vi "09_dosing.vi"() -> ()   [LabVIEW 2024]
uses:
  <vilib>/Utility/error.llb/DialogType.ctl
  4067e6f5-c9bb-441e-8d38-abed3cce061a.vi
  <vilib>/Waveform/WDTOps.llb/WDT Get XY Value DBL.vi
  <vilib>/Utility/file.llb/Write Delimited Spreadsheet (DBL).vi
  <instrlib>/Tektronix DMM40x0 Series/Tektronix DMM40x0 Series.lvlib
panel:
  out "Current Time":timestamp
  out "Current Voltage":dbl format="%0.2f"
  in  "stop":bool
  out "STABLE":bool
  in  "Serial Communication":T1={"Baud Rate"=9600, "Parity"=0, "Data Bits"=8, "Stop Bits"=10, "Flow Control"=0} {"Flow Control" items=["None", "XON/XOFF", "RTS/CTS", "XON/XOFF & RTS/CTS", "DTR/DSR", "XON/XOFF & DTR/DSR"]; "Stop Bits" items=["1.0"=10, "1.5"=15, "2.0"=20]; "Data Bits" items=["7"=7, "8"=8]; "Parity" items=["None", "Odd", "Even", "Mark", "Space"]; "Baud Rate" items=["300"=300, "600"=600, "1200"=1200, "2400"=2400, "4800"=4800, "9600"=9600, "19200"=19200]}
  out "Stability threshold":dbl format="%#_13g"
  out "Waveform Graph":dbl[](graph)
  # "Voltmeter Serial Configuration"
  # "DEFAULT SETTINGS:\n\nTimeout (10000 ms)\nTrigger Count (5000)\nSample Count (1)\n\n****DC VOLTAGE***"
  # "Voltmeter Stability"
  # "0 - Stability threshold not met\n1 - Stability threshold met\n\n\n\n*stability (+/-0.05 mV) of last 15 pts"
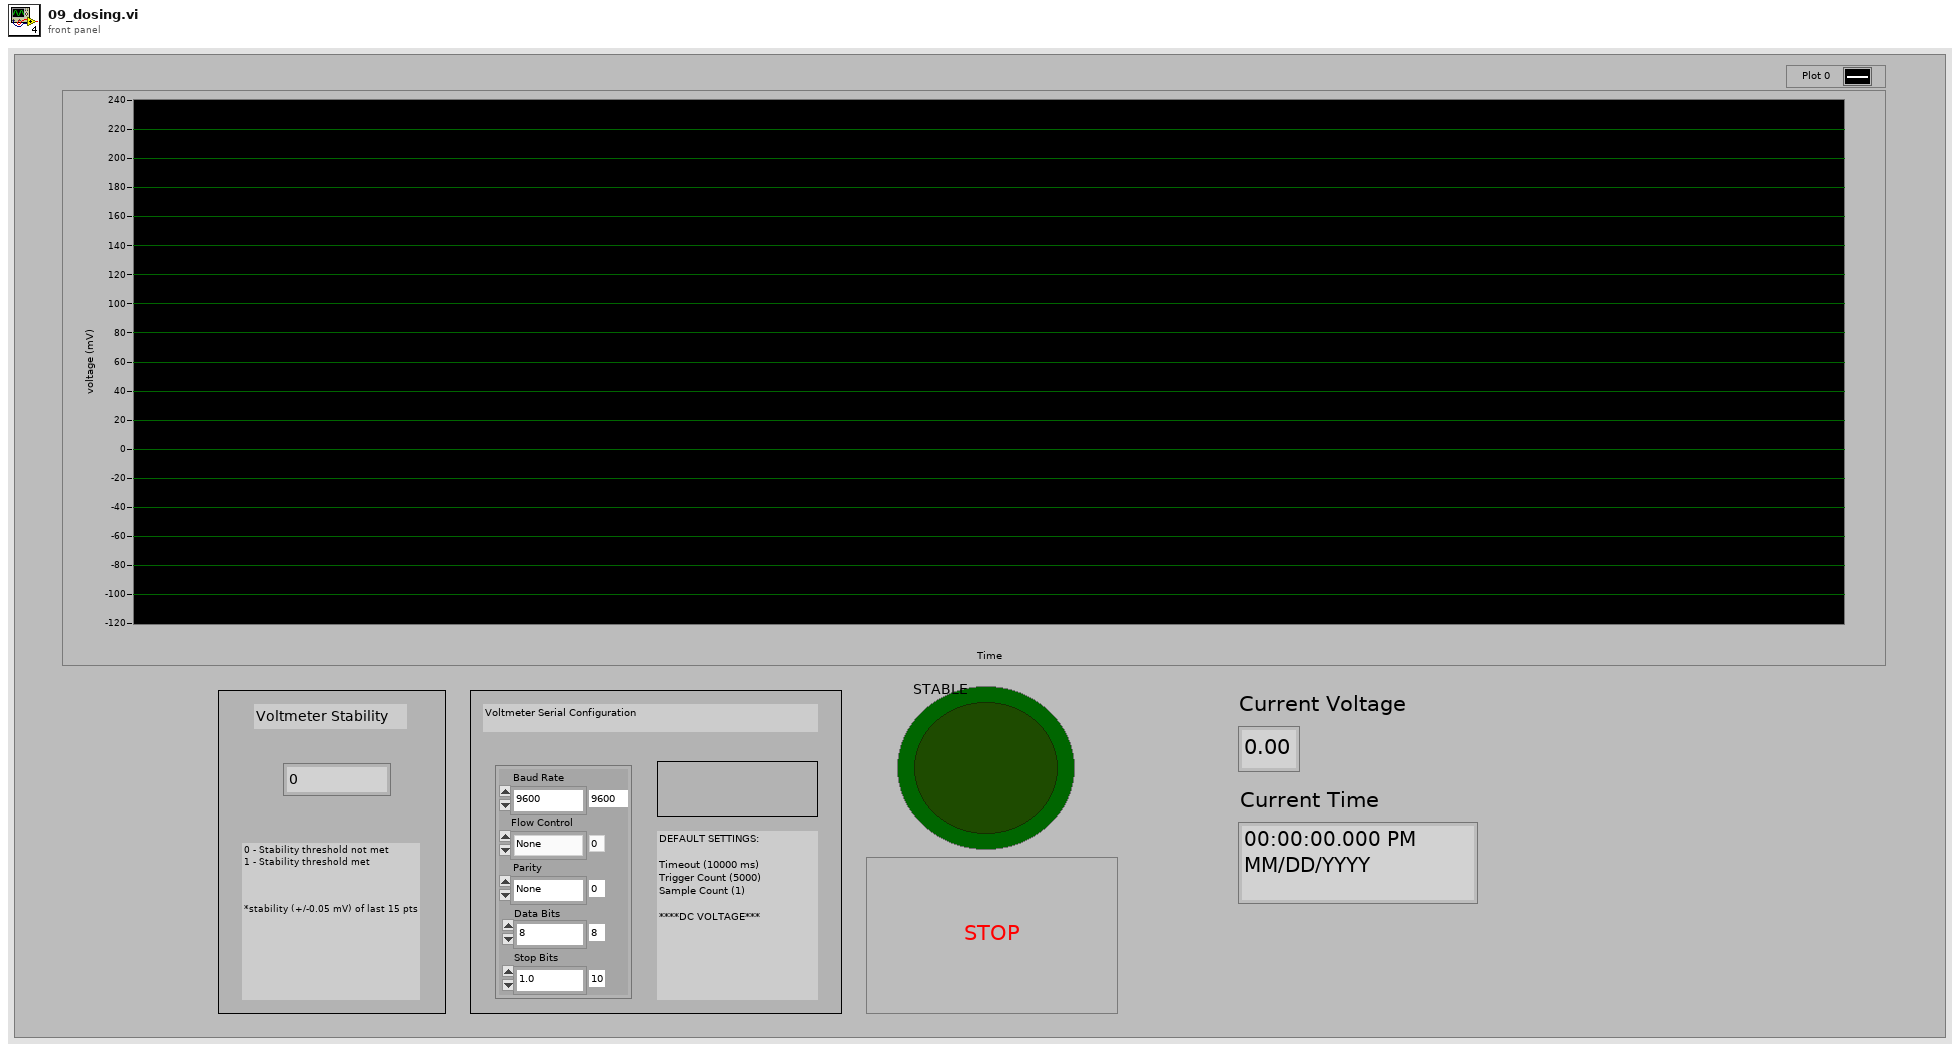
[diagram p1: front panel]
types:
  T1 = cluster{"Baud Rate":u32, "Parity":u16, "Data Bits":u16, "Stop Bits":u16, "Flow Control":u16}
  T2 = typedef "DialogType.ctl" = u16
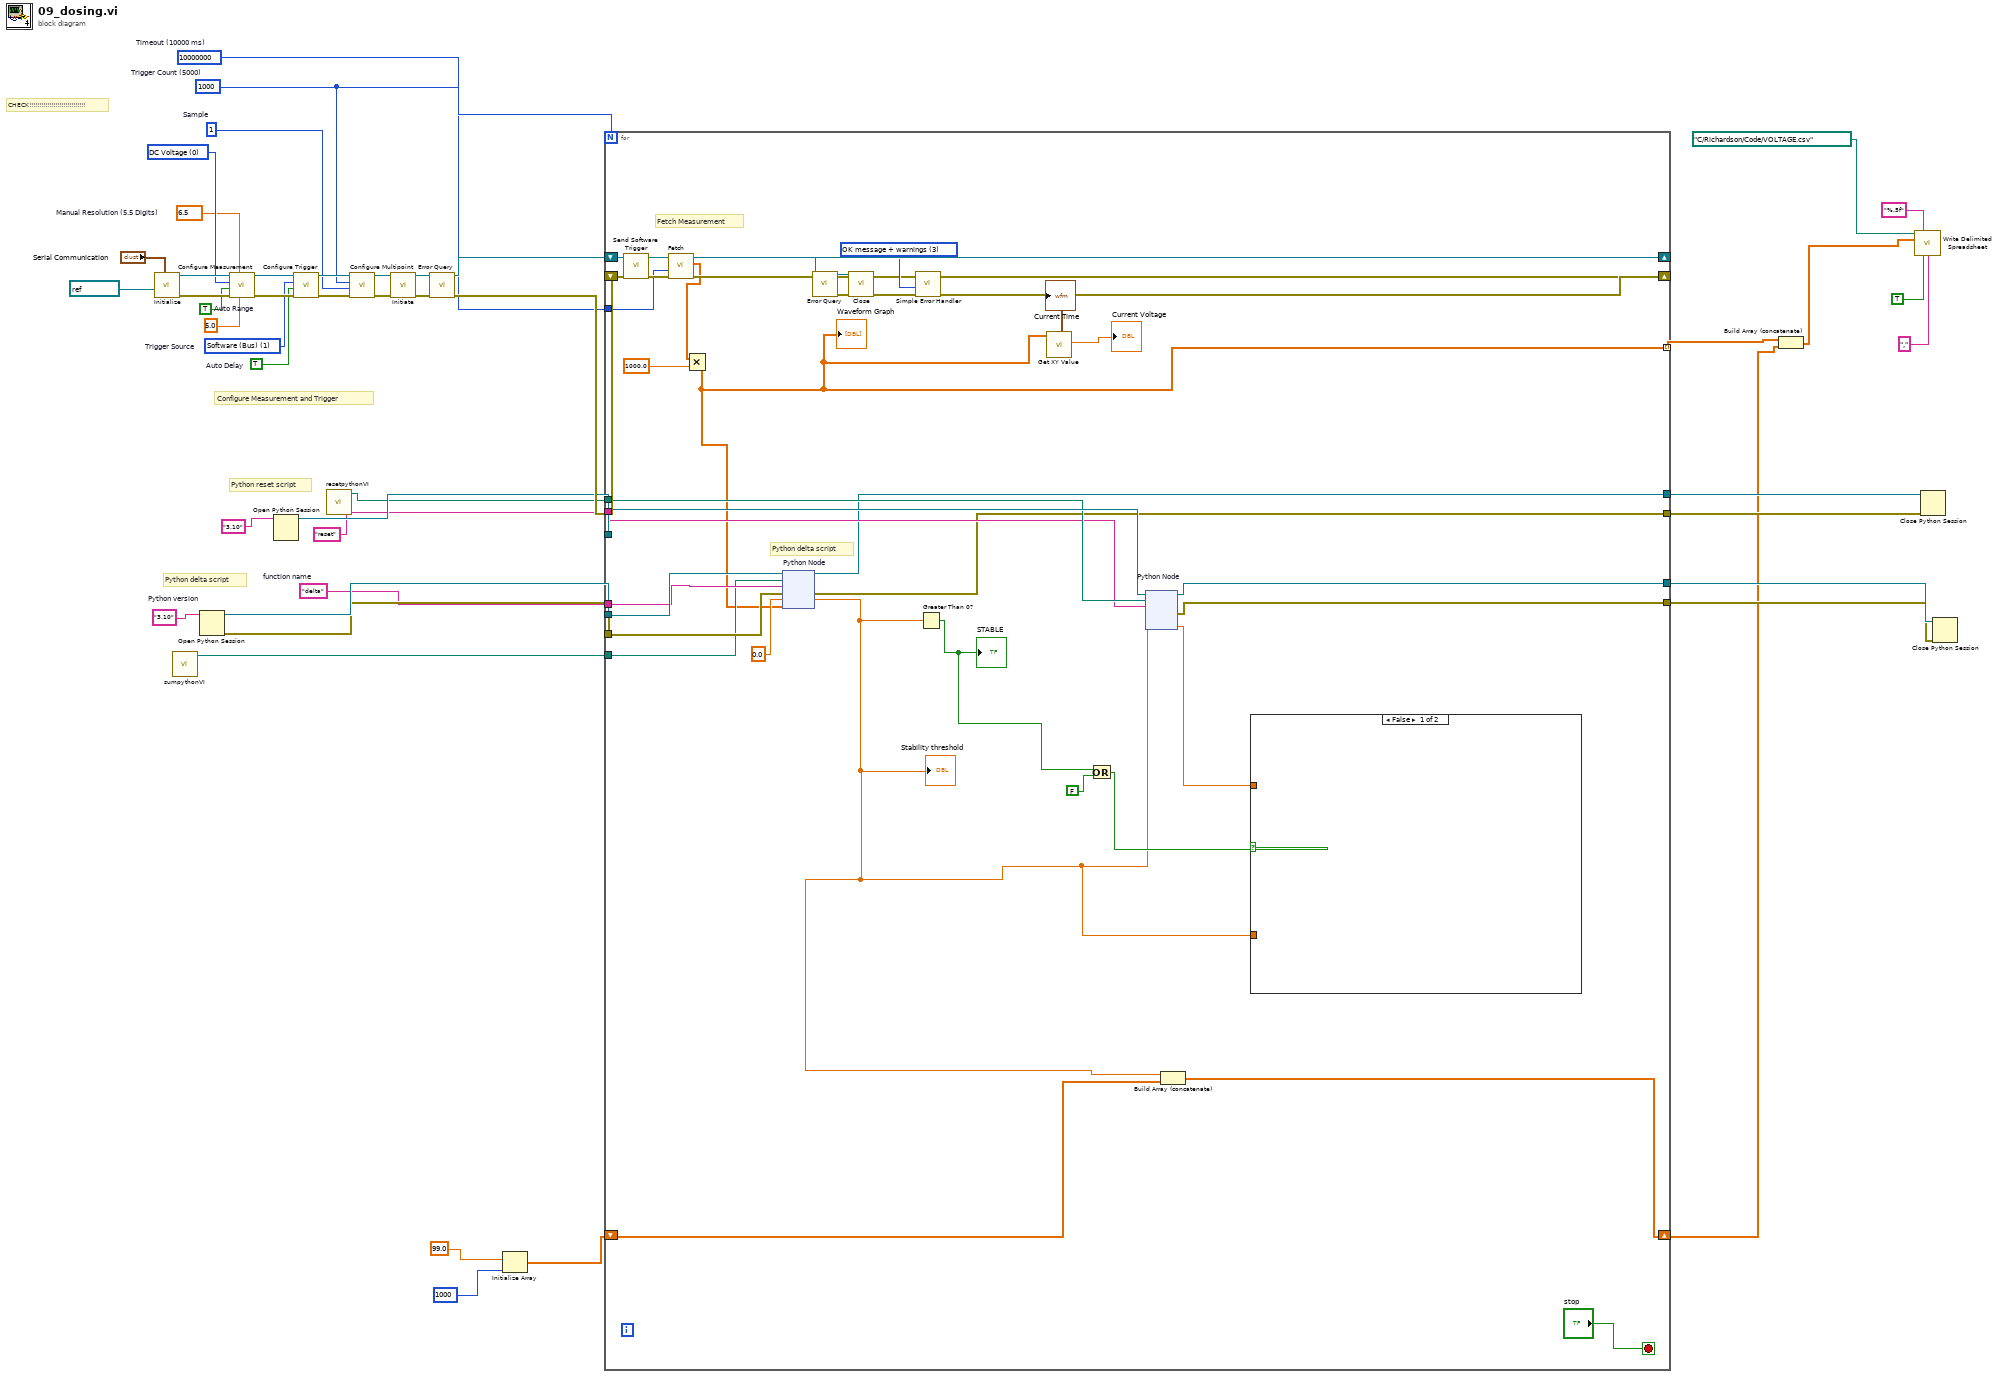
[diagram p0: block diagram]
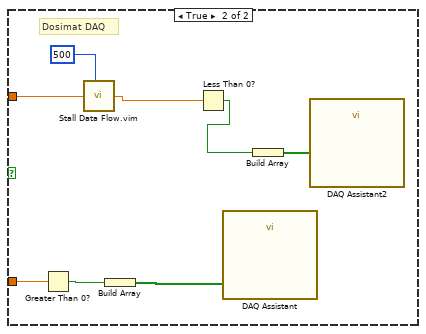
[diagram p2: hidden frame]
diagram:
  w11 = T2 3 items=["no dialog", "OK message", "continue or stop message", "OK message + warnings", "continue/stop + warnings"] ("type of dialog (OK msg:1)")
  w24 = "delta"  # function name
  w27 = "3.10"  # Python version
  w39 = u16 0 items=["DC Voltage", "AC Voltage", "2 - Wire Resistance", "4 - Wire Resistance", "DC Current", "AC Current", "Frequency", "Period", "Continuity", "Diode Checking", "Temperature", "Capacitance"] ("Function (0: DC Voltage)")
  w30 = u32 10000000  # Timeout (10000 ms)
  w31 = 1  # Sample
  w38 = 1000  # Trigger Count (5000)
  w32 = 6.5 items=["4.5"=4.5, "5.5"=5.5, "6.5"=6.5]  # Manual Resolution (5.5 Digits)
  w40 = TRUE  # Auto Delay
  w41 = u16 1 items=["Immediate", "Software (Bus)", "External"]  # Trigger Source
  w42 = TRUE  # Auto Range
  # "Python delta script"
  # "Python reset script"
  # "CHECK!!!!!!!!!!!!!!!!!!!!!!!!!!!!"
  # "Configure Measurement and Trigger"
  n1 = call <instrlib>:"Initialize.vi"("Serial Configuration"="Serial Communication", "VISA resource name"=refnum<visa-resource-name> "COM2" ("COM PORT (COM2)")) -> ("error out"=w51:errorcluster, "VISA resource name out"=w52:refnum<visa-resource-name>)  [unwired: 3 in, 5 out]
  n2 = call "sumpythonVI.vi"() -> ("appended path"=w23:path)  [unwired: 11 in]
  n3 = Open Python Session(python version=w27) -> (session out=w29:refnum<k35>, error out=w28:errorcluster)  [unwired: 2 in]
  n4 = call <instrlib>:"Configure Measurement.vi"("Manual Range (1.0)"=5.0, "Manual Resolution (5.5 Digits)"=w32, "error in (no error)"=w51, "Auto Range (T:Enable)"=w42, "Function (0: DC Voltage)"=w39, "VISA resource name"=w52) -> ("error out"=w49:errorcluster, "VISA resource name out"=w50:refnum<visa-resource-name>)  [unwired: 4 out]
  n5 = Open Python Session(python version="3.10" ("Python version")) -> (session out=w25:refnum<k35>)  [unwired: 2 in, 1 out]
  n6 = call <instrlib>:"Configure Trigger.vi"("error in (no error)"=w49, "Auto Delay (T: Enable)"=w40, "Trigger Source (0: Immediate)"=w41, "VISA resource name"=w50) -> ("error out"=w47:errorcluster, "VISA resource name out"=w48:refnum<visa-resource-name>)  [unwired: 1 in, 5 out]
  n7 = call "resetpythonVI.vi"() -> ("appended path"=w22:path)  [unwired: 11 in]
  n8 = call <instrlib>:"Configure Multipoint.vi"("error in (no error)"=w47, "Sample Count (1)"=w31, "Trigger Count (1)"=w38, "VISA resource name"=w48) -> ("error out"=w45:errorcluster, "VISA resource name out"=w46:refnum<visa-resource-name>)  [unwired: 6 out]
  n9 = call <instrlib>:"Initiate.vi"("error in (no error)"=w45, "VISA resource name"=w46) -> ("error out"=w37:errorcluster, "VISA resource name out"=w36:refnum<visa-resource-name>)  [unwired: 8 out]
  n10 = call <instrlib>:"Error Query.vi"("error in (no error)"=w37, "VISA resource name"=w36) -> ("error out"=w34:errorcluster, "VISA resource name out"=w35:refnum<visa-resource-name>)  [unwired: 8 out]
  n11 = Initialize Array(99.0, 1000 ("dimension size")) -> (w4:dbl[])
  n12 = for {
    N: w38 -> [_]
    shift-right: [w83] -> w13
    shift-left: w34 -> [w79]
    shift-right: [w84] -> w15
    shift-left: w35 -> [w80]
    tunnel: w30 -> [w78]
    tunnel: w29 -> [w73]
    tunnel: w28 -> [w72]
    tunnel: w25 -> [w71]
    tunnel: w24 -> [w70]
    tunnel: w23 -> [w69]
    tunnel: w22 -> [w68]
    tunnel: "reset" ("function name") -> [w67]
    tunnel: [w66] -> w20
    tunnel: [w65] -> w19
    tunnel: [w64] -> w18
    tunnel: [w63] -> w17
    shift-right: [w59] -> w1
    shift-left: w4 -> [w56]
    tunnel: [w55] -> w2 mode=indexing
    stop <- "stop" stop-if-true
    # "Python delta script"
    # "Fetch Measurement"
    n13 = call <instrlib>:"Send Software Trigger.vi"("error in (no error)"=w79, "VISA resource name"=w80) -> ("error out"=w81:errorcluster, "VISA resource name out"=w82:refnum<visa-resource-name>)  [unwired: 8 out]
    n14 = call <instrlib>:"Fetch.vi"("error in (no error)"=w81, "Timeout (10000 ms)"=w78, "VISA resource name"=w82) -> ("error out"=w83:errorcluster, "Measurements"=w76:dbl[], "VISA resource name out"=w84:refnum<visa-resource-name>)  [unwired: 6 out]
    n15 = Multiply(x=w76, y=1000.0) -> (x*y=w55:dbl[])
    "Waveform Graph" <- w55
    n16 = node "Python Node"(w73, w69, w70, w72, 0.0, w55) -> (w64:refnum<k35>, w63:errorcluster, w57:dbl)  [unwired: 1 in, 2 out]
    "Stability threshold" <- w57
    n17 = Greater Than 0?(x=w57) -> (x > 0?=w60:bool)
    "STABLE" <- w60
    n18 = call-poly <vilib>:"Get XY Value.vi"("waveform in"=w55) -> ("actual Y position"=→"Current Voltage":dbl, "X value"=→"Current Time":timestamp)  [unwired: 6 in, 3 out]
    n19 = Or(x=w60, y=FALSE) -> (x .or. y?=w58:bool)
    n20 = node "Python Node"(w71, w68, w67, w57) -> (w66:refnum<k35>, w65:errorcluster, w74:dbl)  [unwired: 3 in, 2 out]
    n21 = Build Array (concatenate)(w57, w56) -> (w59:dbl[])
    n22 = case shown="False" w58 {
      tunnel: w74 -> [_ w87]
      tunnel: w57 -> [_ w85]
      frame False {
      }
      frame True {
        # "Dosimat DAQ"
        n23 = Greater Than 0?(x=w85) -> (x > 0?=w90:bool)
        n24 = call "Stall Data Flow.vim"("value in"=w87, "milliseconds to wait"=u32 500) -> ("value out"=w88:dbl)  [unwired: 1 out]
        n25 = Build Array(w90) -> (w89:bool[])
        n26 = Less Than 0?(x=w88) -> (x < 0?=w91:bool)
        n27 = call "DAQ Assistant"("data"=w89) -> ()  [unwired: 17 in, 2 out]
        n28 = Build Array(w91) -> (w92:bool[])
        n29 = call "DAQ Assistant2"("data"=w92) -> ()  [unwired: 17 in, 2 out]
      }
    }
  }
  n30 = call <instrlib>:"Error Query.vi"("error in (no error)"=w13, "VISA resource name"=w15) -> ("error out"=w12:errorcluster, "VISA resource name out"=w14:refnum<visa-resource-name>)  [unwired: 8 out]
  n31 = call <instrlib>:"Close.vi"("error in (no error)"=w12, "VISA resource name"=w14) -> ("error out"=w16:errorcluster)  [unwired: 9 out]
  n32 = call <vilib>:"Simple Error Handler.vi"("type of dialog (OK msg:1)"=w11, "error in (no error)"=w16) -> ()  [unwired: 8 out]
  n33 = Build Array (concatenate)(w2, w1) -> (w3:dbl[][])
  n34 = call-poly <vilib>:"Write Delimited Spreadsheet.vi"("file path (dialog if empty)"=path "C:/Richardson/Code/VOLTAGE.csv", "format (%.3f)"="%.5f", "2D data"=w3, "transpose? (no:F)"=TRUE, "delimiter (\\t)"="," ("delimiter (\\t)")) -> ()  [unwired: 9 in, 2 out]
  n35 = Close Python Session(session in=w18, error in=w17) -> ()  [unwired: 1 out]
  n36 = Close Python Session(session in=w20, error in=w19) -> ()  [unwired: 1 out]
